vi "Add Object.vi"(8 "error in":errorcluster, 10 "element":refnum<class>, 11 "Buffer in":refnum<data-value>) -> (0 "error out":errorcluster, 1 "overflowed":bool, 2 "overflow":refnum<class>, 3 "Buffer":refnum<data-value>)   [LabVIEW 2013, in "CircularBuffer.lvlib" / "ObjectBuffer.lvclass"]
doc: "This VI writes one data element into the current location in the buffer. The location in the buffer is updated automatically."
uses:
  ObjectBuffer.lvclass
  VariantBuffer/VariantBuffer.lvclass
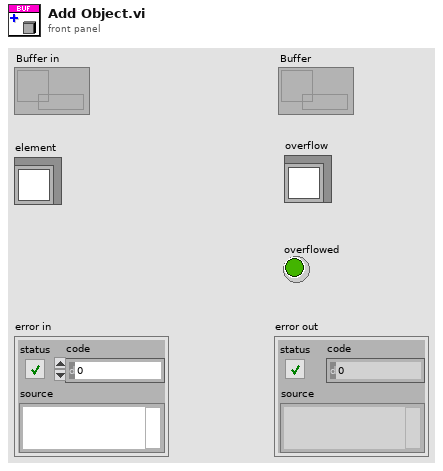
[diagram p1: front panel]
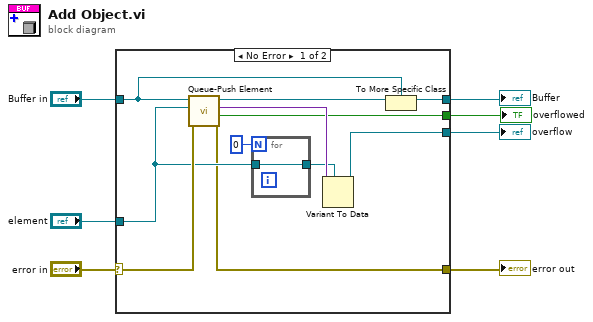
[diagram p0: block diagram]
diagram:
  n1 = case shown="No Error" "error in" {
    selector: "error in" -> [w17 w21]
    tunnel: "Buffer in" -> [w15 w20]
    tunnel: [w16 w20] -> w6
    tunnel: [w8 w21] -> w3
    tunnel: "element" -> [w13 _]
    tunnel: [w12 _] -> w2
    tunnel: [w9 _] -> w1
    frame No Error {
      n2 = call "Queue-Push Element.vi"("error in"=w17, "element"=w13, "Buffer in"=w15) -> ("error out"=w8:errorcluster, "overflowed"=w9:bool, "overflow"=w11:variant, "Buffer"=w18:refnum<data-value>)  [unwired: 5 in]
      n3 = for {
        N: 0 -> [_]
        tunnel: w13 -> [w19]
        tunnel: [w19] -> w10
      }
      n4 = Variant To Data(type=w10, Variant=w11) -> (data=w12:refnum<class>)  [unwired: 1 in, 1 out]
      n5 = To More Specific Class(target class=w15, reference=w18) -> (specific class reference=w16:refnum<data-value>)  [unwired: 1 in, 1 out]
    }
    frame Error {
    }
  }
  "error out" <- w3
  "Buffer" <- w6
  "overflow" <- w2
  "overflowed" <- w1
